vi "RSZVB Query Verification Sweep Results.vi"(8 "error in (no error)":errorcluster {"code" format="%.0x"}, 11 "VISA session":refnum<visa-resource-name>) -> (0 "error out":errorcluster {"code" format="%.0x"}, 1 "Max Offset":dbl format="%^.3e", 2 "Calibration Passed":bool, 3 "dup VISA session":refnum<visa-resource-name>)   [LabVIEW 2011]
doc: "This VI returns the result of the last verification sweep. \n\nNote(s):\n\n(1) For some measurements the default set timeout can be insufficient. To set higher timeout use VI rszvb_setTimeOut.\n\n(2) This VI requires an enabled verification sweep - set with VI rszvb_SetVerificationSweepState.\n\n(3) If no verification sweep result is available, the VI returns RSZVB_ERROR_INSTRUMENT_DATA_NOT_AVAILABLE.\n\nRemote-control command(s):\nSOURce<Ch>:POWer<Pt>:CORRection[:ACQuire]:VERification:RESult?"
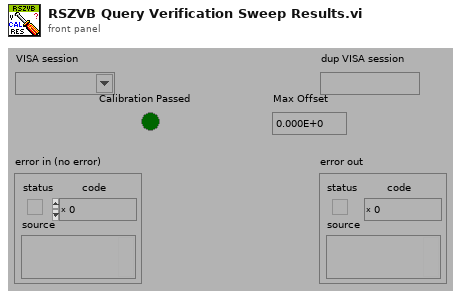
[diagram p1: front panel]
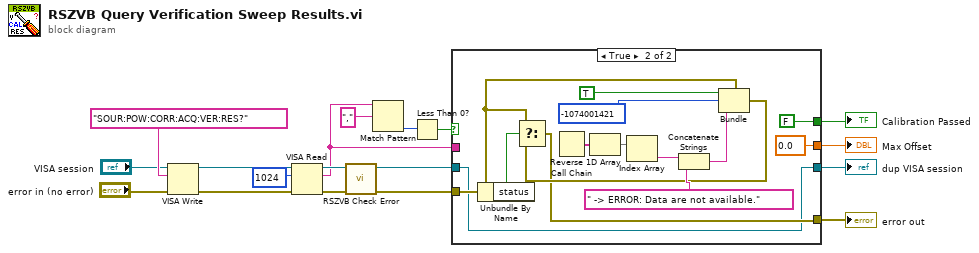
[diagram p0: block diagram]
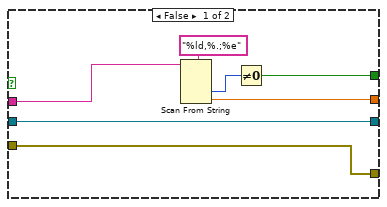
[diagram p2: hidden frame]
diagram:
  n1 = VISA Write(VISA resource name="VISA session", write buffer="SOUR:POW:CORR:ACQ:VER:RES?", error in (no error)="error in (no error)") -> (VISA resource name out=w15:refnum<visa-resource-name>, error out=w14:errorcluster)  [unwired: 1 out]
  n2 = VISA Read(VISA resource name=w15, byte count=u32 1024 ("byte count (0)"), error in (no error)=w14) -> (VISA resource name out=w17:refnum<visa-resource-name>, read buffer=w3:string, error out=w16:errorcluster)  [unwired: 1 out]
  n3 = call "RSZVB Check Error.vi"("error in (no error)"=w16, "VISA session"=w17) -> ("error out"=w8:errorcluster, "dup VISA session"=w5:refnum<visa-resource-name>)  [unwired: 8 in]
  n4 = Match Pattern(string=w3, regular expression=",") -> (offset past match=w9:i32)  [unwired: 1 in, 3 out]
  n5 = Less Than 0?(x=w9) -> (x < 0?=w6:bool)
  n6 = case shown="True" w6 {
    tunnel: w8 -> [w24 w30]
    tunnel: [w24 w29] -> w7
    tunnel: w5 -> [w25 w28]
    tunnel: [w25 w28] -> w4
    tunnel: w3 -> [w21 _]
    tunnel: [w20 0.0] -> w2
    tunnel: [w19 FALSE] -> w1
    frame False {
      n7 = Scan From String(format string="%ld,%.;%e", input string=w21) -> (output 1=w23:i32, output 2=w20:dbl)  [unwired: 4 in, 3 out]
      n8 = Not Equal To 0?(x=w23) -> (x != 0?=w19:bool)
    }
    frame True {
      n9 = Unbundle By Name(w30) -> ("status"=w32:bool)
      n10 = Call Chain() -> (call chain=w35:string[])
      n11 = Reverse 1D Array(array=w35) -> (reversed array=w36:string[])
      n12 = Index Array(array=w36) -> (element=w37:string)  [unwired: 1 in]
      n13 = Concatenate Strings(w37, " -> ERROR: Data are not available." ("string")) -> (w39:string)
      n14 = Bundle(cluster=w30, "status"=TRUE, "code"=-1074001421, "source"=w39) -> (w31:errorcluster)
      n15 = Select(t=w30, s=w32, f=w31) -> (s? t:f=w29:errorcluster)
    }
  }
  "error out" <- w7
  "dup VISA session" <- w4
  "Calibration Passed" <- w1
  "Max Offset" <- w2
